vi "ReceiveData_Sub.vi"(8 "error in (no error)":errorcluster, 11 "LabVIEW-Python-Interface in":refnum<class "PyLVi.lvclass">) -> (0 "error out":errorcluster, 1 "return list":T1[](array[typedef]), 3 "LabVIEW-Python-Interface out":refnum<class "PyLVi.lvclass">)   [LabVIEW 2016, in "PyLVi.lvlib" / "PyLVi.lvclass"]
uses:
  PyLVi.lvclass
  Controls/ArgumentStructure.ctl
  Controls/DescriptorStructure.ctl
  PyLVi.lvclass/PyLVi.ctl
  <vilib>/addons/zeromq/zmq_socket.lvclass
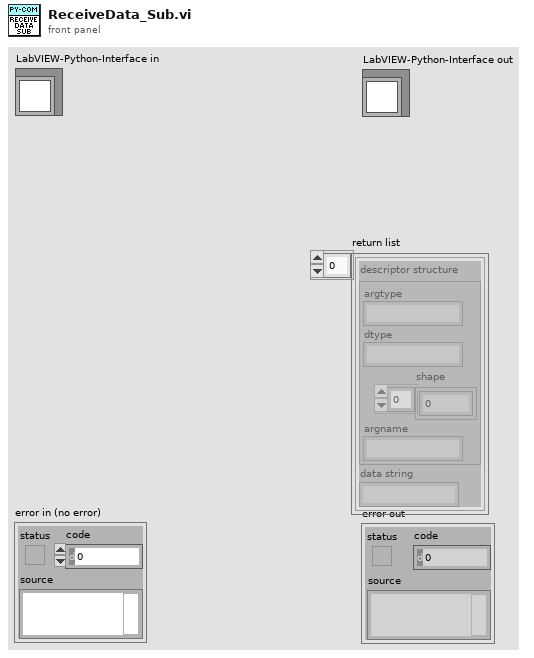
[diagram p1: front panel]
types:
  T1 = typedef "PyLVi.lvlib/PyLVi.lvclass/ArgumentStructure.ctl" = cluster{"descriptor structure":T2, "data string":string}
  T2 = typedef "PyLVi.lvlib/PyLVi.lvclass/DescriptorStructure.ctl" = cluster{"argtype":string, "dtype":string, "shape":u32[], "argname":string}
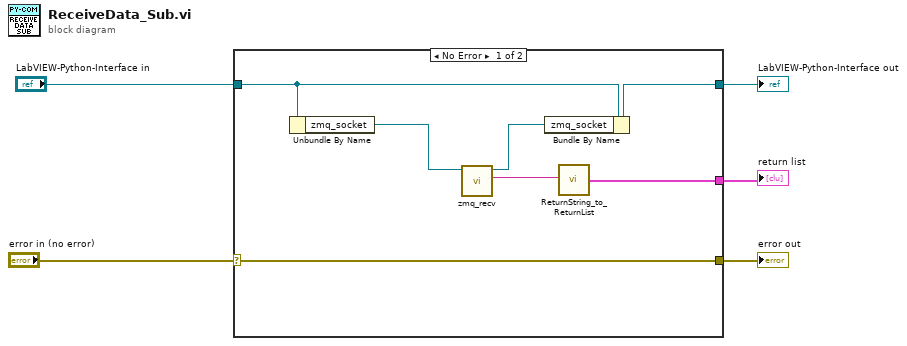
[diagram p0: block diagram]
diagram:
  n1 = case shown="No Error" "error in (no error)" {
    selector: "error in (no error)" -> [w12 w13]
    tunnel: [w12 w13] -> w4
    tunnel: [w10 w14] -> w2
    tunnel: "LabVIEW-Python-Interface in" -> [w11 w14]
    tunnel: [w6 _] -> w1
    frame No Error {
      n2 = Unbundle By Name(w11) -> ("zmq_socket"=w9:refnum<class "zmq_socket.lvclass">)
      n3 = call <vilib>:"zmq_recv.vi"("socket in"=w9) -> ("data"=w7:string, "socket out"=w8:refnum<class "zmq_socket.lvclass">)  [unwired: 4 in, 3 out]
      n4 = Bundle By Name(cluster=w11, "zmq_socket"=w8) -> (w10:refnum<class "PyLVi.lvclass">)
      n5 = call "ReturnString_to_ReturnList.vi"("return string"=w7) -> ("return list"=w6:T1[])  [unwired: 3 in, 1 out]
    }
    frame Error {
    }
  }
  "error out" <- w4
  "LabVIEW-Python-Interface out" <- w2
  "return list" <- w1
